vi "Flock_Master_IncrementRev.vi"(8 "error in (no error)":errorcluster) -> (0 "error out":errorcluster)   [LabVIEW 2014, in "FA_Agent_BuildRevision.lvlib"]
uses:
  FA_Agent_BuildRevision.lvlib
panel:
  in  "Cancel Button":bool
  out "IterationNum":i32
  in  "IterationNum":i32
  in  "Build":bool
  in  "BuildNum":i32
  in  "MinorRev":i32
  in  "MajorRev":i32
  out "BuildNum":i32
  out "MinorRev":i32
  out "MajorRev":i32
  in  "configuration file path":path=path "C:/Users/Mark Black/Perforce/penguin_1666/mblack_PerforceWin/user/mblack/FlockAgent/trunk/Agent/source/Static Source/FA_Config.ini"
  # "Previous Build"
  # "New Build"
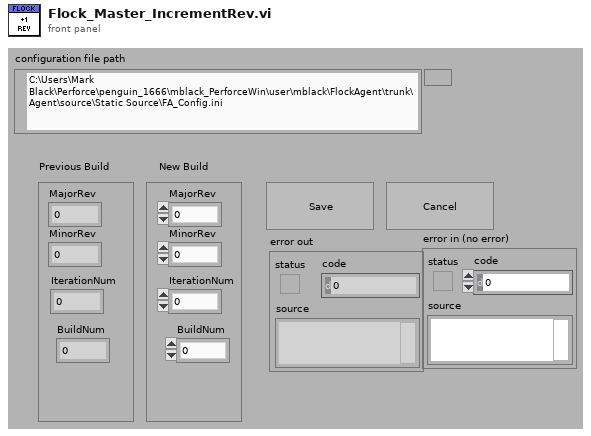
[diagram p1: front panel]
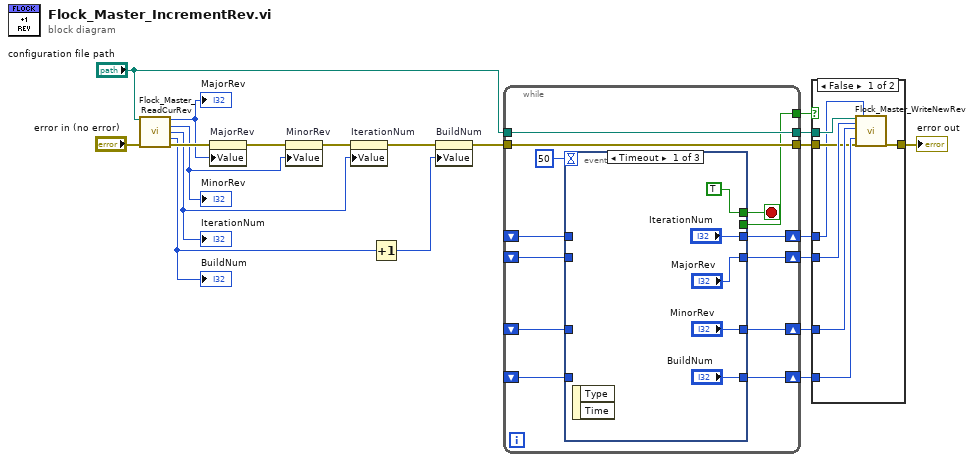
[diagram p0: block diagram]
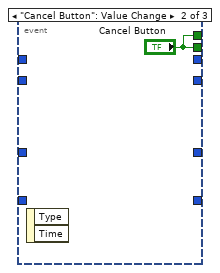
[diagram p3: hidden frame]
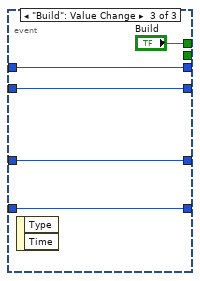
[diagram p4: hidden frame]
diagram:
  n1 = call "Flock_Master_ReadCurRev.vi"("configuration file path"="configuration file path", "error in (no error)"="error in (no error)") -> ("MajorRev"=w8:i32, "MinorRev"=w9:i32, "IterationNum"=w1:i32, "BuildNum"=w10:i32, "error out"=w12:errorcluster)  [unwired: 9 in]
  "MajorRev" <- w8
  "MinorRev" <- w9
  "BuildNum" <- w10
  "IterationNum" <- w1
  n2 = property on="MajorRev" class="DigNum (strict)"(error in=w12, "Value"=w8) -> (error out=w20:errorcluster)  [unwired: 1 in, 1 out]
  n3 = property on="MinorRev" class="DigNum (strict)"(error in=w20, "Value"=w9) -> (error out=w6:errorcluster)  [unwired: 1 in, 1 out]
  n4 = property on="IterationNum" class="DigNum (strict)"(error in=w6, "Value"=w1) -> (error out=w2:errorcluster)  [unwired: 1 in, 1 out]
  n5 = Increment(x=w10) -> (x+1=w18:i32)
  n6 = property on="BuildNum" class="DigNum (strict)"(error in=w2, "Value"=w18) -> (error out=w19:errorcluster)  [unwired: 1 in, 1 out]
  n7 = while {
    tunnel: w19 -> [w28]
    tunnel: "configuration file path" -> [w33]
    tunnel: [w33] -> w17
    tunnel: [w28] -> w13
    shift-right: [w31] -> w16
    shift-left: _ -> [w25]
    shift-right: [w30] -> w15
    shift-left: _ -> [w26]
    shift-right: [w29] -> w14
    shift-left: _ -> [w27]
    shift-right: [w24] -> w7
    shift-left: _ -> [w23]
    tunnel: [w21] -> w5
    stop <- w22 stop-if-true
    n8 = event shown="[0] Timeout" {
      selector: _ -> [_ _ _]
      dyn-events: _ -> [_ _ _]
      timeout: 50 ("Numeric") -> [_ _ _]
      tunnel: [TRUE ("Build") "Cancel Button" "Build"] -> w22
      tunnel: ["MajorRev" _ w41] -> w31
      tunnel: ["MinorRev" _ w42] -> w30
      tunnel: ["BuildNum" _ w43] -> w29
      tunnel: w27 -> [_ _ w43]
      tunnel: w26 -> [_ _ w42]
      tunnel: w25 -> [_ _ w41]
      tunnel: ["IterationNum" _ w40] -> w24
      tunnel: w23 -> [_ _ w40]
      tunnel: [_ "Cancel Button" _] -> w21
      event Timeout {
        n9 = event-data() -> ()  [unwired: 1 in, 2 out]
      }
      event "Cancel Button": Value Change {
        n10 = event-data() -> ()  [unwired: 1 in, 2 out]
      }
      event "Build": Value Change {
        n11 = event-data() -> ()  [unwired: 1 in, 2 out]
      }
    }
  }
  n12 = case shown="False" w5 {
    tunnel: w17 -> [w51 _]
    tunnel: w16 -> [w50 _]
    tunnel: w15 -> [w49 _]
    tunnel: w14 -> [w48 _]
    tunnel: w13 -> [w47 w52]
    tunnel: w7 -> [w46 _]
    tunnel: [w45 w52] -> w4
    frame False {
      n13 = call "Flock_Master_WriteNewRev.vi"("configuration file path"=w51, "MajorRev"=w50, "MinorRev"=w49, "BuildNum"=w48, "error in (no error)"=w47, "IterationNum"=w46) -> ("error out"=w45:errorcluster)  [unwired: 13 in]
    }
    frame True {
    }
  }
  "error out" <- w4
